vi "TextToLines_jkism++.vi"(6 "Remove Empty Lines?(T)":bool=TRUE, 8 "error in (no error)":errorcluster, 11 "string":string) -> (0 "error out":errorcluster, 3 "Lines":string[](array[string]))   [LabVIEW 2014]
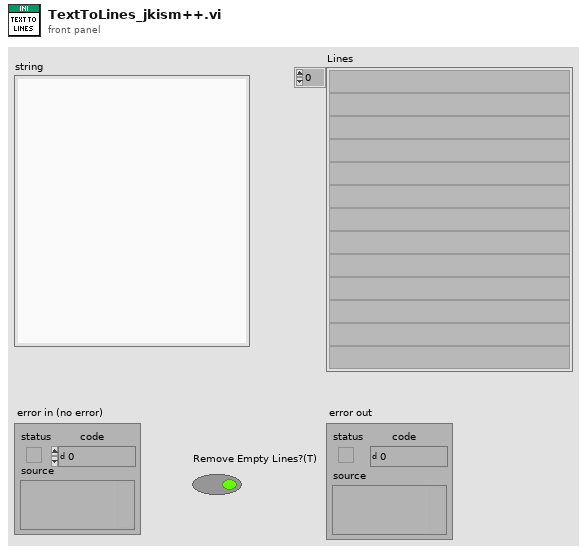
[diagram p1: front panel]
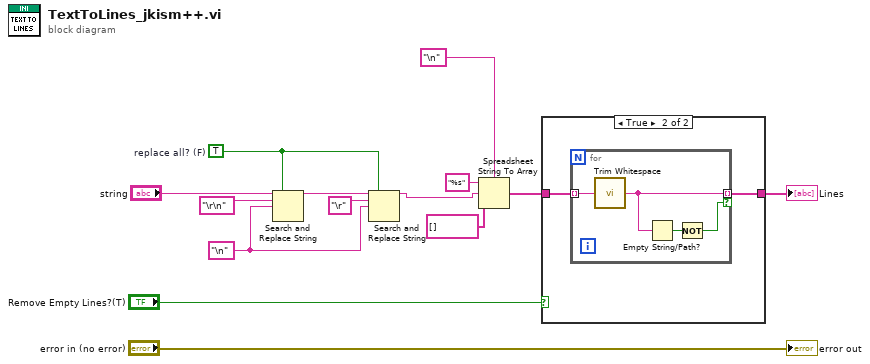
[diagram p0: block diagram]
diagram:
  w6 = TRUE  # replace all? (F)
  w7 = "\n" ("delimiter (Tab)")
  n1 = Search and Replace String(replace all?=w6, input string="string", search string="\r\n" ("delimiter (Tab)"), replace string=w7) -> (result string=w10:string)  [unwired: 4 in, 3 out]
  n2 = Search and Replace String(replace all?=w6, input string=w10, search string="\r" ("delimiter (Tab)"), replace string=w7) -> (result string=w8:string)  [unwired: 4 in, 3 out]
  n3 = Spreadsheet String To Array(delimiter (Tab)="\n", format string="%s", spreadsheet string=w8, array type (2D Dbl)=string[] [] ("Array of Strings")) -> (array=w11:string[])
  n4 = case shown="True" "Remove Empty Lines?(T)" {
    tunnel: [w15 w17] -> w13
    tunnel: w11 -> [w15 w16]
    frame False {
    }
    frame True {
      n5 = for {
        tunnel: w16 -> [w21] mode=indexing
        tunnel: [w20] -> w17 mode=indexing if=w18
        n6 = call <vilib>:"Trim Whitespace.vi"("string"=w21) -> ("trimmed string"=w20:string)  [unwired: 1 in]
        n7 = Empty String/Path?(string/path=w20) -> (empty?=w19:bool)
        n8 = Not(x=w19) -> (.not. x?=w18:bool)
      }
    }
  }
  "Lines" <- w13
  "error out" <- "error in (no error)"
